vi "Add VI to Polymorphic.vi"(8 "error in (no error)":errorcluster, 9 "Polymorphic Label":string, 10 "Path":path, 11 "Polymorphic VI Refnum In":refnum<vi>) -> (0 "error out":errorcluster, 3 "Polymorphic VI Refnum Out":refnum<vi>)   [LabVIEW 2020]
doc: "Adds a VI to a polymorphic VI, applying the Polymorphic Label to the selector. If it already exists in the polymorphic VI, no updates are made."
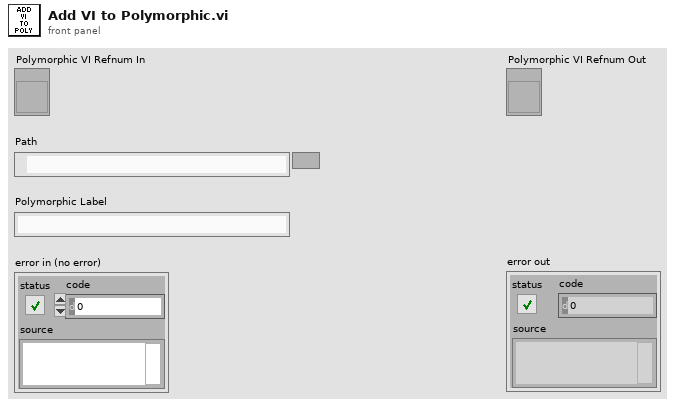
[diagram p1: front panel]
types:
  T1 = cluster{"VIPath":path, "Menu Name":string, "Selector Name":string}[]
  T2 = cluster{"VIPath":path, "Menu Name":string, "Selector Name":string}
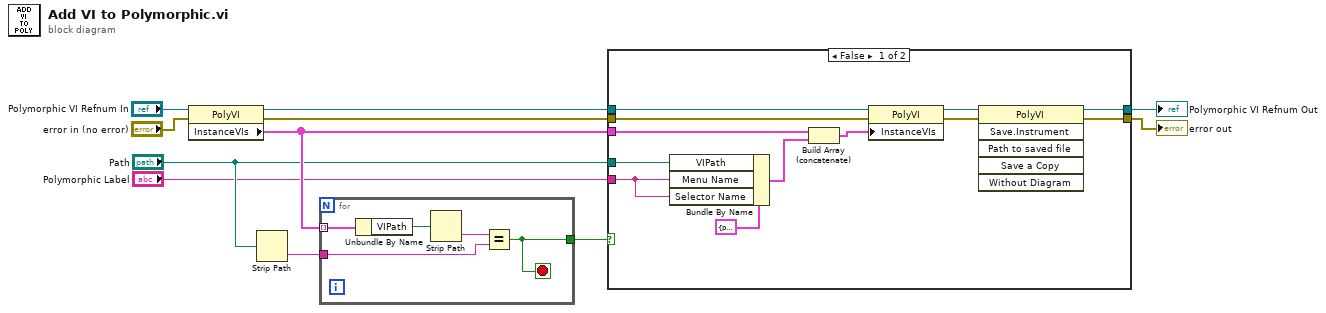
[diagram p0: block diagram]
diagram:
  n1 = property class="PolyVI"(reference="Polymorphic VI Refnum In", error in="error in (no error)") -> (reference out=w8:refnum<vi>, error out=w3:errorcluster, "InstanceVIs"=w9:T1)
  n2 = Strip Path(path="Path") -> (name=w10:string)  [unwired: 1 out]
  n3 = for {
    tunnel: w9 -> [w16] mode=indexing
    tunnel: w10 -> [w13]
    tunnel: [w12] -> w1
    stop <- w12 stop-if-true
    n4 = Unbundle By Name(w16) -> ("VIPath"=w15:path)
    n5 = Strip Path(path=w15) -> (name=w14:string)  [unwired: 1 out]
    n6 = Equal?(x=w14, y=w13) -> (x = y?=w12:bool)
  }
  n7 = case shown="False" w1 {
    tunnel: w9 -> [w27 _]
    tunnel: w8 -> [w28 w30]
    tunnel: "Path" -> [w24 _]
    tunnel: "Polymorphic Label" -> [w23 _]
    tunnel: [w20 w30] -> w5
    tunnel: w3 -> [w19 w29]
    tunnel: [w17 w29] -> w2
    frame False {
      n8 = Bundle By Name(cluster=T2 {"VIPath"=path "", "Menu Name"="", "Selector Name"=""}, "VIPath"=w24, "Menu Name"=w23, "Selector Name"=w23) -> (w22:T2)
      n9 = Build Array (concatenate)(w27, w22) -> (w25:T1)
      n10 = property class="PolyVI"(reference=w28, error in=w19, "InstanceVIs"=w25) -> (reference out=w21:refnum<vi>, error out=w18:errorcluster)
      n11 = invoke class="PolyVI" method="Save.Instrument"(reference=w21, error in=w18) -> (reference out=w20:refnum<vi>, error out=w17:errorcluster)  [unwired: 4 in, 4 out]
    }
    frame True {
    }
  }
  "Polymorphic VI Refnum Out" <- w5
  "error out" <- w2
